vi "LUCS001RT_Navigation1.vi"(8 "error in (no error)":errorcluster, 11 "NavParam":T1={"Lat1Hem"=33.0, "Lat1Rad"=57.0, "Lon1Hem"=0.0, "Lon1Rad"=0.0, "Lat2Hem"=118.0, "Lat2Rad"=24.0, "Lon2Hem"=0.0, "Lon2Rad"=0.0, "DistanceRad"=40.0, "DistanceNM"=38.0, "CourseCond"=0.0, "TrueCourseRad"=0.0, "LatDegCurr"=73, "LatMinCurr"=47.0, "LatHemCurr"=0.0, "LatRadCurr"=0.0, "LonDegCurr"=0, "LonMinCurr"=0.0, "LonHemCurr"=0.0, "LonRadCurr"=-0.7023601432666094, "XTD"=40.0, "DistCurrRad"=38.0, "TrueCourseCurrRad"=0.0, "DistCurrNM"=0.7091854527270293, "TrueCourseDeg"=73.0, "TrueCourseCurrDeg"=47.0, "LON1"=0.0, "LAT1"=1.2877620997631494, "LON2"=38.0, "LAT2"=38.0} {"DistanceNM" format="%#.3f"}) -> (0 "error out":errorcluster, 3 "NavParamOut":T1={"Lat1Hem"=33.0, "Lat1Rad"=57.0, "Lon1Hem"=0.0, "Lon1Rad"=0.5925392810520749, "Lat2Hem"=118.0, "Lat2Rad"=24.0, "Lon2Hem"=0.0, "Lon2Rad"=2.066469834361286, "DistanceRad"=40.0, "DistanceNM"=38.0, "CourseCond"=0.0, "TrueCourseRad"=0.7091854527270293, "LatDegCurr"=73, "LatMinCurr"=47.0, "LatHemCurr"=0.0, "LatRadCurr"=1.2877620997631494, "LonDegCurr"=1, "LonMinCurr"=2143.726101388629, "LonHemCurr"=-0.7023601432666094, "LonRadCurr"=-0.7023601432666094, "XTD"=40.0, "DistCurrRad"=38.0, "TrueCourseCurrRad"=0.0, "DistCurrNM"=0.7091854527270293, "TrueCourseDeg"=73.0, "TrueCourseCurrDeg"=47.0, "LON1"=0.0, "LAT1"=1.2877620997631494, "LON2"=38.0, "LAT2"=38.0} {"DistanceNM" format="%#.3f"})   [LabVIEW 2020]
uses:
  TypeDefs/NavigationParams.ctl
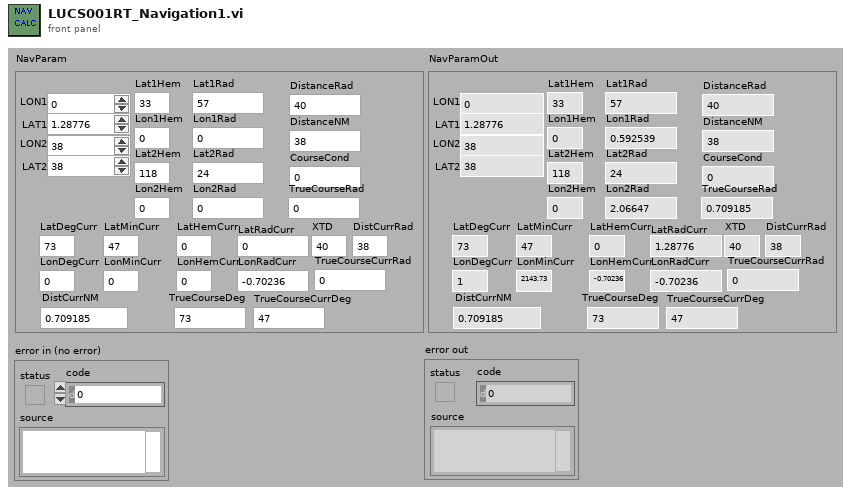
[diagram p1: front panel]
types:
  T1 = typedef "NavigationParams.ctl" = cluster{"Lat1Hem":dbl, "Lat1Rad":dbl, "Lon1Hem":dbl, "Lon1Rad":dbl, "Lat2Hem":dbl, "Lat2Rad":dbl, "Lon2Hem":dbl, "Lon2Rad":dbl, "DistanceRad":dbl, "DistanceNM":dbl, "CourseCond":dbl, "TrueCourseRad":dbl, "LatDegCurr":i32, "LatMinCurr":dbl, "LatHemCurr":dbl, "LatRadCurr":dbl, "LonDegCurr":i32, "LonMinCurr":dbl, "LonHemCurr":dbl, "LonRadCurr":dbl, "XTD":dbl, "DistCurrRad":dbl, "TrueCourseCurrRad":dbl, "DistCurrNM":dbl, "TrueCourseDeg":dbl, "TrueCourseCurrDeg":dbl, "LON1":dbl, "LAT1":dbl, "LON2":dbl, "LAT2":dbl}
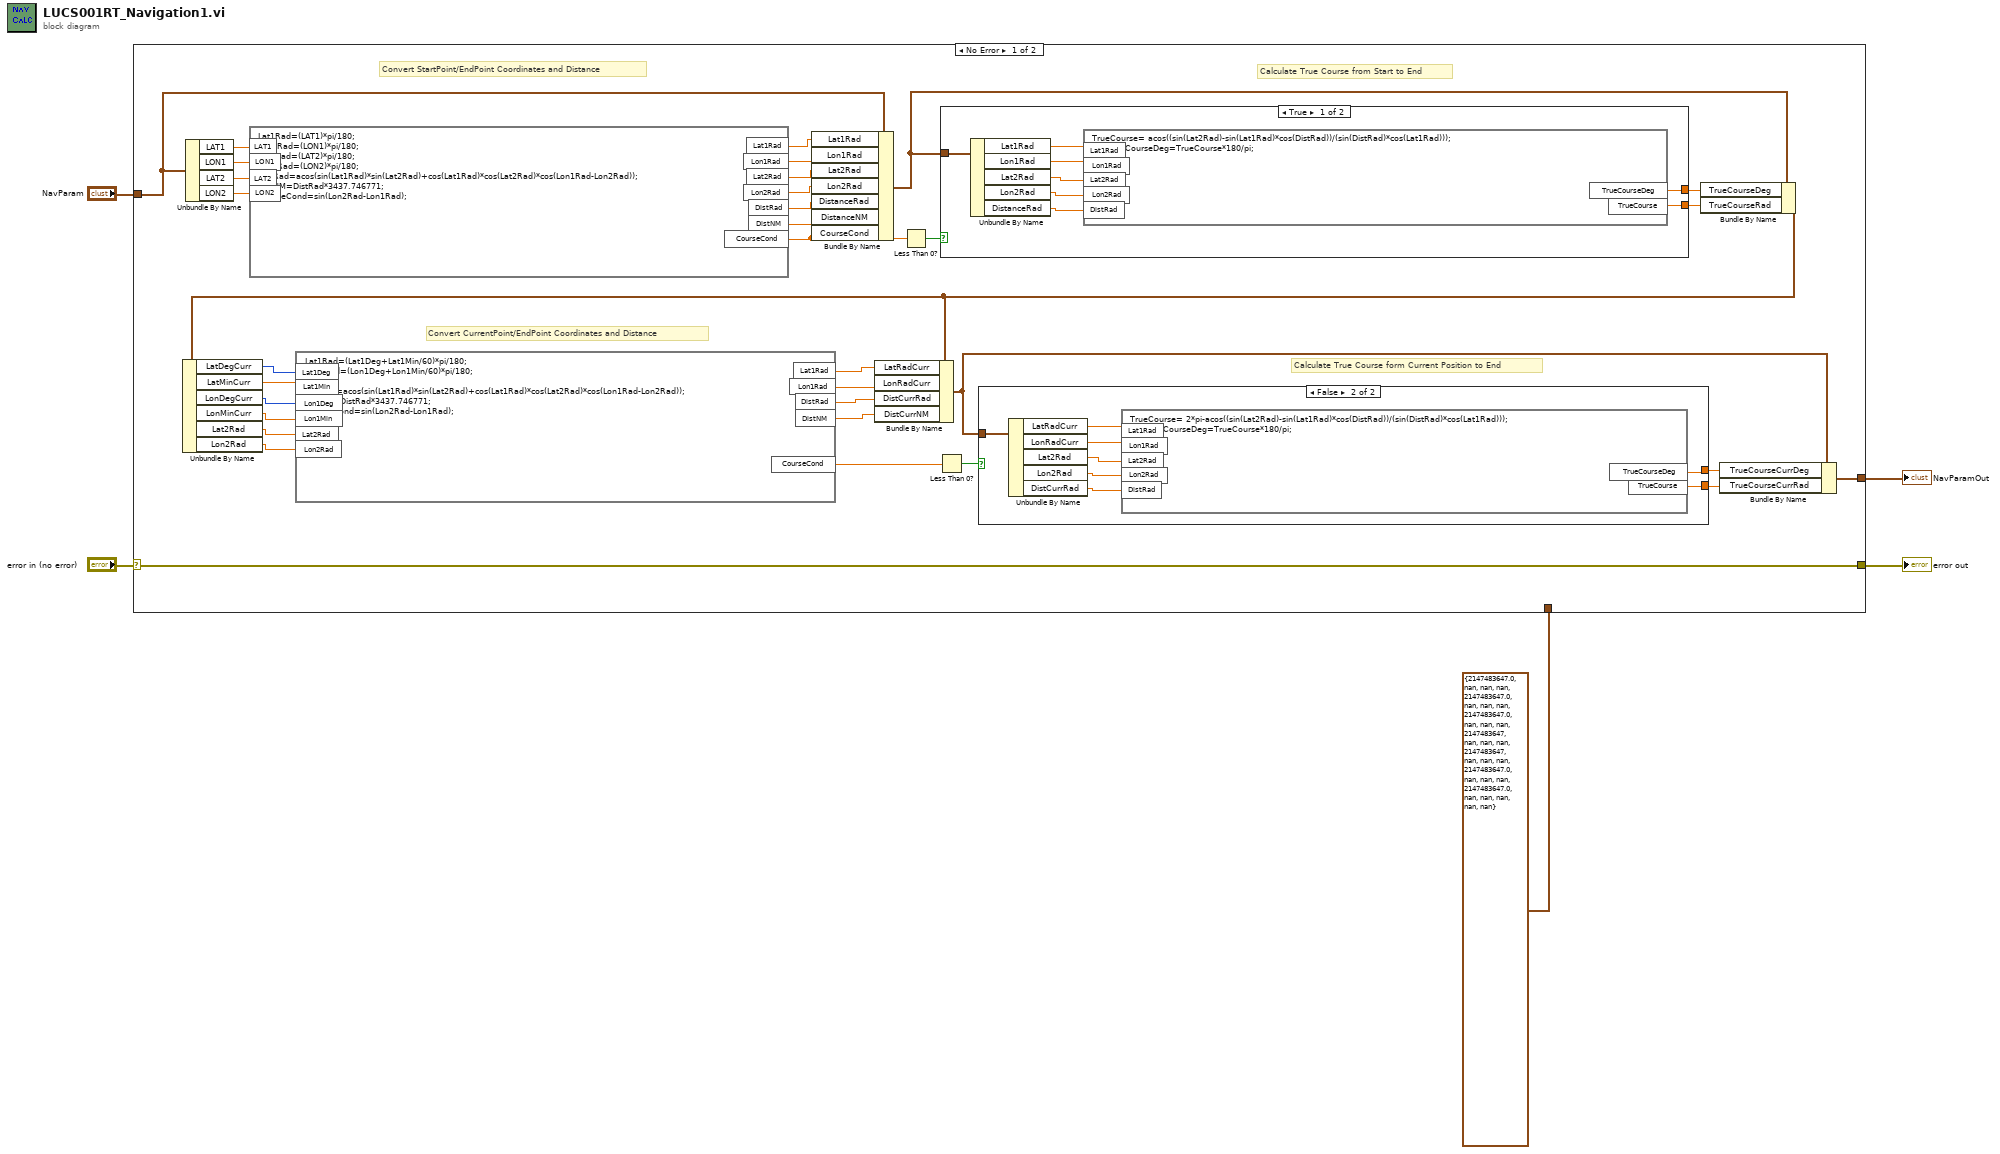
[diagram p0: block diagram]
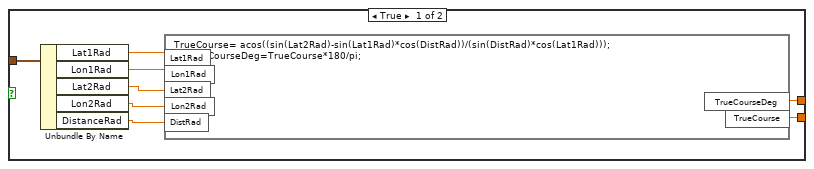
[diagram p2: hidden frame]
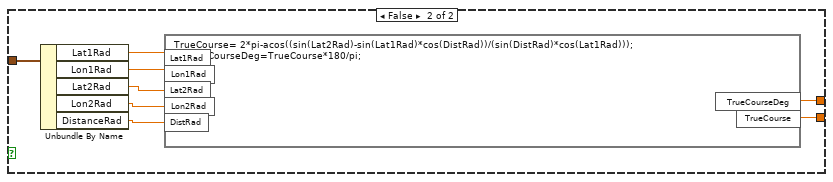
[diagram p3: hidden frame]
diagram:
  n1 = case shown="No Error" "error in (no error)" {
    selector: "error in (no error)" -> [w6 w73]
    tunnel: "NavParam" -> [w35 _]
    tunnel: [w11 w72] -> w4
    tunnel: [w6 w73] -> w2
    tunnel: T1 {"Lat1Hem"=2147483647.0, "Lat1Rad"=nan, "Lon1Hem"=nan, "Lon1Rad"=nan, "Lat2Hem"=2147483647.0, "Lat2Rad"=nan, "Lon2Hem"=nan, "Lon2Rad"=nan, "DistanceRad"=2147483647.0, "DistanceNM"=nan, "CourseCond"=nan, "TrueCourseRad"=nan, "LatDegCurr"=2147483647, "LatMinCurr"=nan, "LatHemCurr"=nan, "LatRadCurr"=nan, "LonDegCurr"=2147483647, "LonMinCurr"=nan, "LonHemCurr"=nan, "LonRadCurr"=nan, "XTD"=2147483647.0, "DistCurrRad"=nan, "TrueCourseCurrRad"=nan, "DistCurrNM"=nan, "TrueCourseDeg"=2147483647.0, "TrueCourseCurrDeg"=nan, "LON1"=nan, "LAT1"=nan, "LON2"=nan, "LAT2"=nan} ("NavParam") -> [_ w72]
    frame No Error {
      # "Convert CurrentPoint/EndPoint Coordinates and Distance"
      # "Calculate True Course form Current Position to End"
      # "Calculate True Course from Start to End"
      # "Convert StartPoint/EndPoint Coordinates and Distance"
      n2 = Unbundle By Name(w35) -> ("LAT1"=w39:dbl, "LON1"=w38:dbl, "LAT2"=w37:dbl, "LON2"=w36:dbl)
      n3 = formula code="Lat1Rad=(LAT1)*pi/180;\nLon1Rad=(LON1)*pi/180;\nLat2Rad=(LAT2)*pi/180;\nLon2Rad=(LON2)*pi/180;\nDistRad=acos(sin(Lat1Rad)*sin(Lat2Rad)+cos(Lat1Rad)*cos(Lat2Rad)*cos(Lon1Rad-Lon2Rad));\nDistNM=DistRad*3437.746771;\nCourseCond=sin(Lon2Rad-Lon1Rad);"("LAT1"=w39, "LON1"=w38, "LAT2"=w37, "LON2"=w36) -> ("Lat1Rad"=w34:dbl, "Lon1Rad"=w33:dbl, "Lat2Rad"=w32:dbl, "Lon2Rad"=w31:dbl, "DistRad"=w30:dbl, "DistNM"=w29:dbl, "CourseCond"=w7:dbl)
      n4 = Bundle By Name(cluster=w35, "Lat1Rad"=w34, "Lon1Rad"=w33, "Lat2Rad"=w32, "Lon2Rad"=w31, "DistanceRad"=w30, "DistanceNM"=w29, "CourseCond"=w7) -> (w27:T1)
      n5 = Less Than 0?(x=w7) -> (x < 0?=w28:bool)
      n6 = case shown="True" w28 {
        tunnel: w27 -> [w63 w71]
        tunnel: [w57 w65] -> w26
        tunnel: [w56 w64] -> w9
        frame True {
          n7 = Unbundle By Name(w63) -> ("Lat1Rad"=w62:dbl, "Lon1Rad"=w61:dbl, "Lat2Rad"=w60:dbl, "Lon2Rad"=w59:dbl, "DistanceRad"=w58:dbl)
          n8 = formula code="TrueCourse= acos((sin(Lat2Rad)-sin(Lat1Rad)*cos(DistRad))/(sin(DistRad)*cos(Lat1Rad)));\n     TrueCourseDeg=TrueCourse*180/pi;"("Lat1Rad"=w62, "Lon1Rad"=w61, "Lat2Rad"=w60, "Lon2Rad"=w59, "DistRad"=w58) -> ("TrueCourse"=w57:dbl, "TrueCourseDeg"=w56:dbl)
        }
        frame False {
          n9 = Unbundle By Name(w71) -> ("Lat1Rad"=w70:dbl, "Lon1Rad"=w69:dbl, "Lat2Rad"=w68:dbl, "Lon2Rad"=w67:dbl, "DistanceRad"=w66:dbl)
          n10 = formula code="TrueCourse= 2*pi-acos((sin(Lat2Rad)-sin(Lat1Rad)*cos(DistRad))/(sin(DistRad)*cos(Lat1Rad)));\n    TrueCourseDeg=TrueCourse*180/pi;"("Lat1Rad"=w70, "Lon1Rad"=w69, "Lat2Rad"=w68, "Lon2Rad"=w67, "DistRad"=w66) -> ("TrueCourse"=w65:dbl, "TrueCourseDeg"=w64:dbl)
        }
      }
      n11 = Bundle By Name(cluster=w27, "TrueCourseDeg"=w9, "TrueCourseRad"=w26) -> (w19:T1)
      n12 = Unbundle By Name(w19) -> ("LatDegCurr"=w25:i32, "LatMinCurr"=w24:dbl, "LonDegCurr"=w23:i32, "LonMinCurr"=w22:dbl, "Lat2Rad"=w21:dbl, "Lon2Rad"=w20:dbl)
      n13 = formula code="Lat1Rad=(Lat1Deg+Lat1Min/60)*pi/180;\nLon1Rad=(Lon1Deg+Lon1Min/60)*pi/180;\n\nDistRad=acos(sin(Lat1Rad)*sin(Lat2Rad)+cos(Lat1Rad)*cos(Lat2Rad)*cos(Lon1Rad-Lon2Rad));\nDistNM=DistRad*3437.746771;\nCourseCond=sin(Lon2Rad-Lon1Rad);"("Lat1Deg"=w25, "Lat1Min"=w24, "Lon1Deg"=w23, "Lon1Min"=w22, "Lat2Rad"=w21, "Lon2Rad"=w20) -> ("Lat1Rad"=w18:dbl, "Lon1Rad"=w17:dbl, "DistRad"=w16:dbl, "DistNM"=w15:dbl, "CourseCond"=w10:dbl)
      n14 = Bundle By Name(cluster=w19, "LatRadCurr"=w18, "LonRadCurr"=w17, "DistCurrRad"=w16, "DistCurrNM"=w15) -> (w12:T1)
      n15 = Less Than 0?(x=w10) -> (x < 0?=w13:bool)
      n16 = case shown="False" w13 {
        tunnel: w12 -> [w47 w55]
        tunnel: [w41 w49] -> w14
        tunnel: [w40 w48] -> w8
        frame True {
          n17 = Unbundle By Name(w47) -> ("Lat1Rad"=w46:dbl, "Lon1Rad"=w45:dbl, "Lat2Rad"=w44:dbl, "Lon2Rad"=w43:dbl, "DistanceRad"=w42:dbl)
          n18 = formula code="TrueCourse= acos((sin(Lat2Rad)-sin(Lat1Rad)*cos(DistRad))/(sin(DistRad)*cos(Lat1Rad)));\n    TrueCourseDeg=TrueCourse*180/pi;"("Lat1Rad"=w46, "Lon1Rad"=w45, "Lat2Rad"=w44, "Lon2Rad"=w43, "DistRad"=w42) -> ("TrueCourse"=w41:dbl, "TrueCourseDeg"=w40:dbl)
        }
        frame False {
          n19 = Unbundle By Name(w55) -> ("LatRadCurr"=w54:dbl, "LonRadCurr"=w53:dbl, "Lat2Rad"=w52:dbl, "Lon2Rad"=w51:dbl, "DistCurrRad"=w50:dbl)
          n20 = formula code="TrueCourse= 2*pi-acos((sin(Lat2Rad)-sin(Lat1Rad)*cos(DistRad))/(sin(DistRad)*cos(Lat1Rad)));\n     TrueCourseDeg=TrueCourse*180/pi;"("Lat1Rad"=w54, "Lon1Rad"=w53, "Lat2Rad"=w52, "Lon2Rad"=w51, "DistRad"=w50) -> ("TrueCourse"=w49:dbl, "TrueCourseDeg"=w48:dbl)
        }
      }
      n21 = Bundle By Name(cluster=w12, "TrueCourseCurrDeg"=w8, "TrueCourseCurrRad"=w14) -> (w11:T1)
    }
    frame Error {
    }
  }
  "NavParamOut" <- w4
  "error out" <- w2
